vi "LDA2_Safety.vi"(1 "Adam Loop Count":i32, 2 "Ch Names":string[](array[string]), 3 "Values":dbl[](array[numeric]) format="%.2f") -> (0 "Scan comment":string)   [LabVIEW 2015]
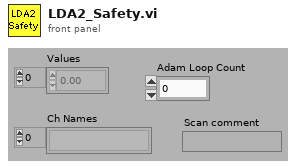
[diagram p1: front panel]
types:
  T1 = typedef "LVDateTimeRec.ctl" = cluster{"fractional second":dbl, "second":i32, "minute":i32, "hour":i32, "day of month":i32, "month":i32, "year":i32, "day of week":i32, "day of year":i32, "DST":i32}
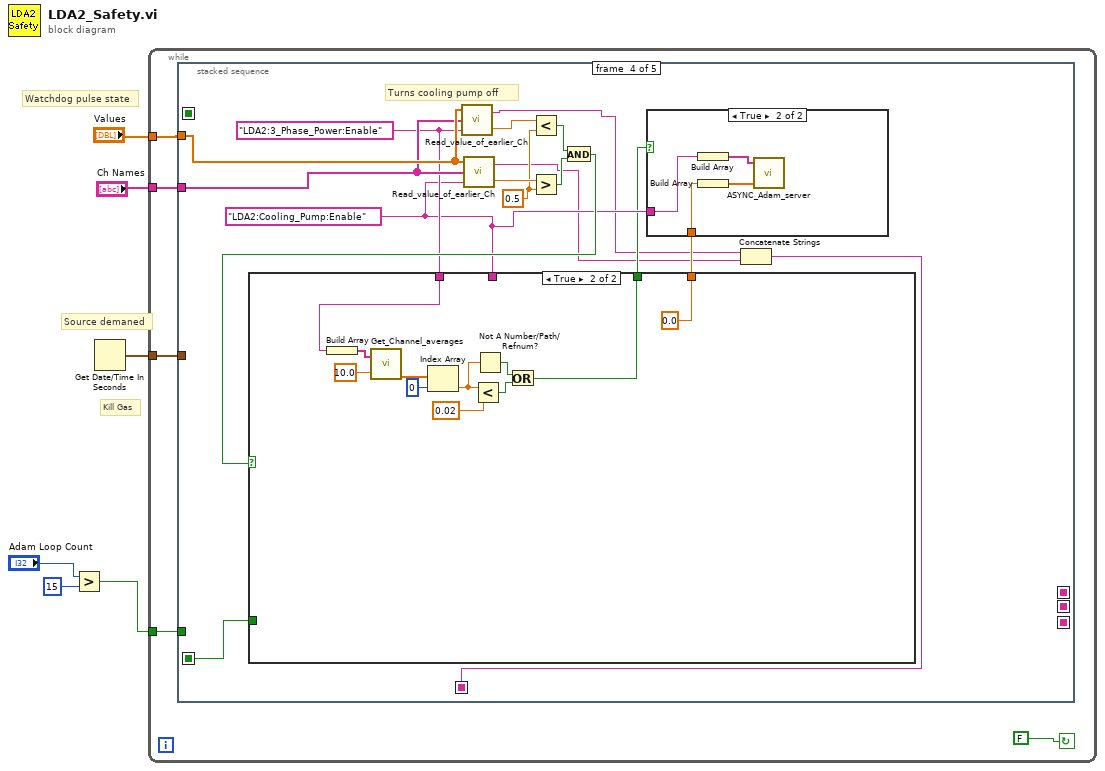
[diagram p0: block diagram]
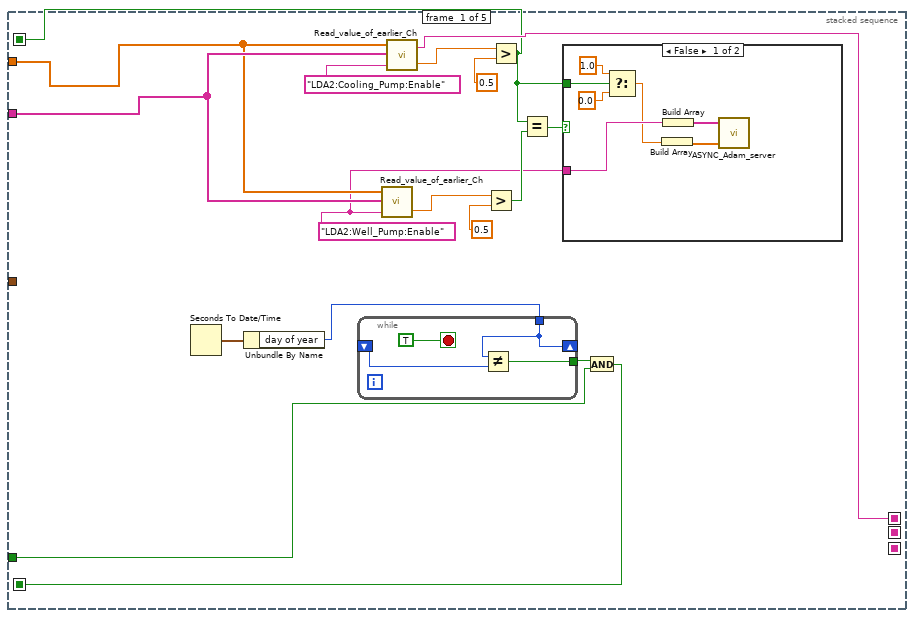
[diagram p2: hidden frame]
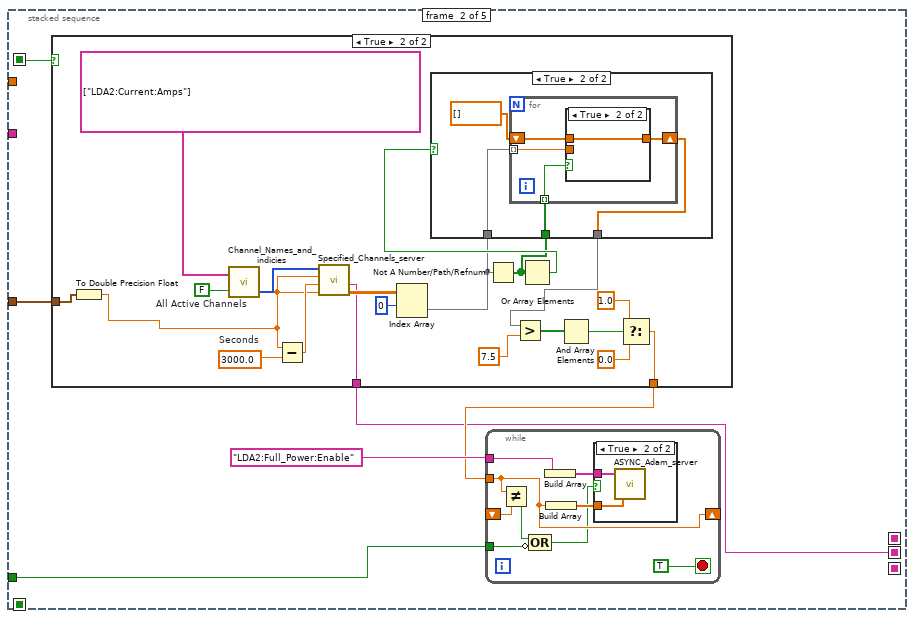
[diagram p4: hidden frame]
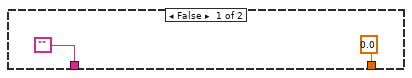
[diagram p6: hidden frame]
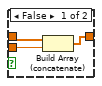
[diagram p8: hidden frame]
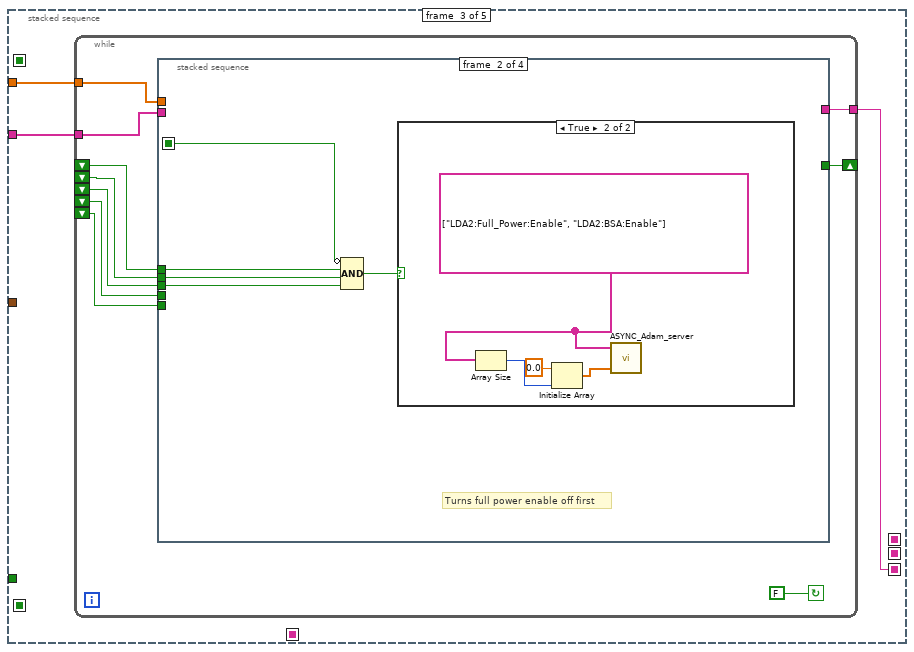
[diagram p9: hidden frame]
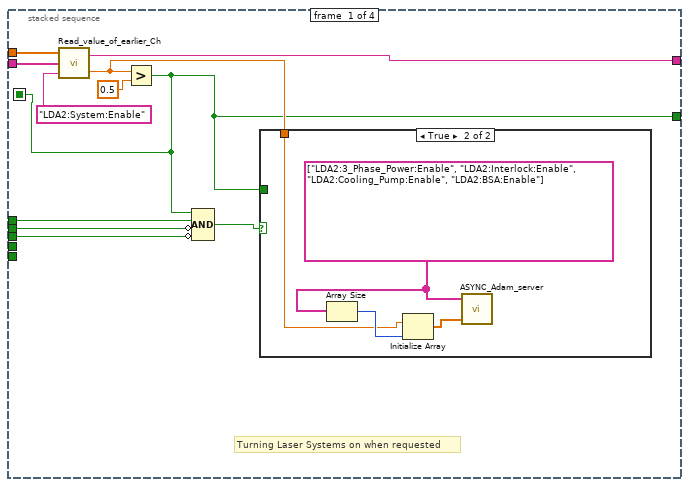
[diagram p10: hidden frame]
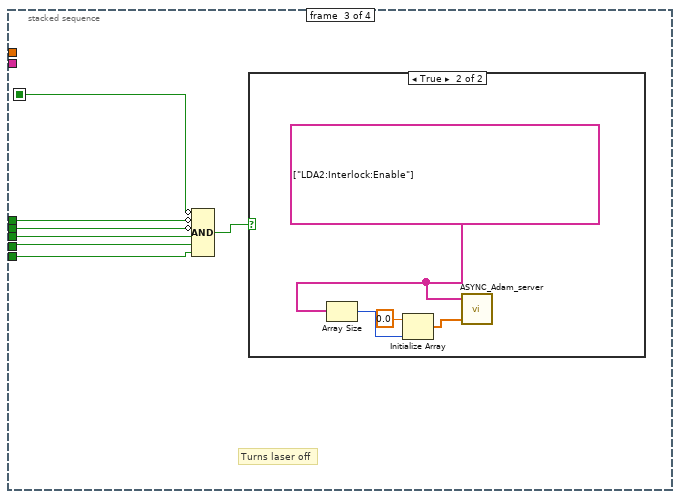
[diagram p13: hidden frame]
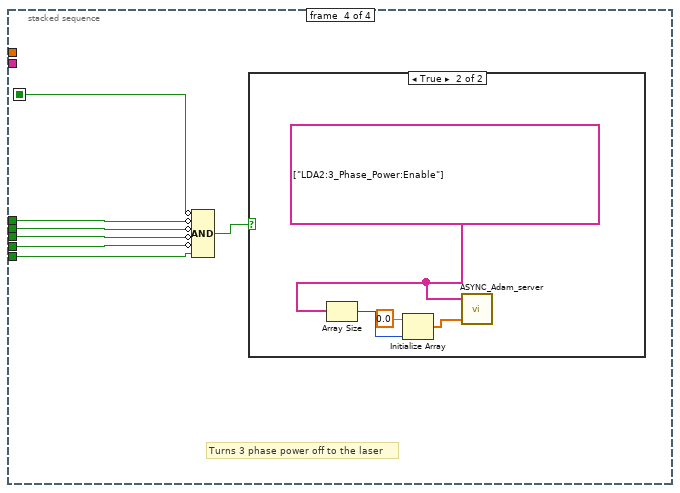
[diagram p15: hidden frame]
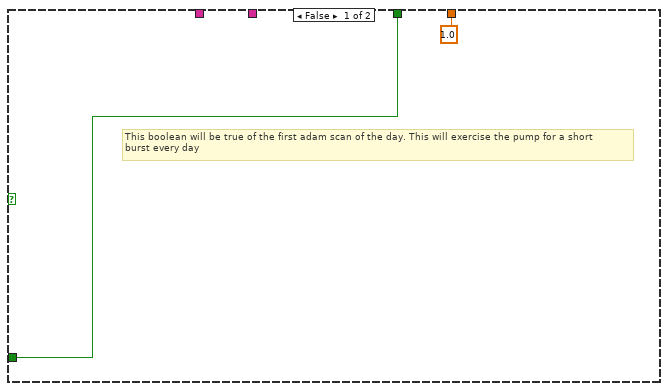
[diagram p18: hidden frame]
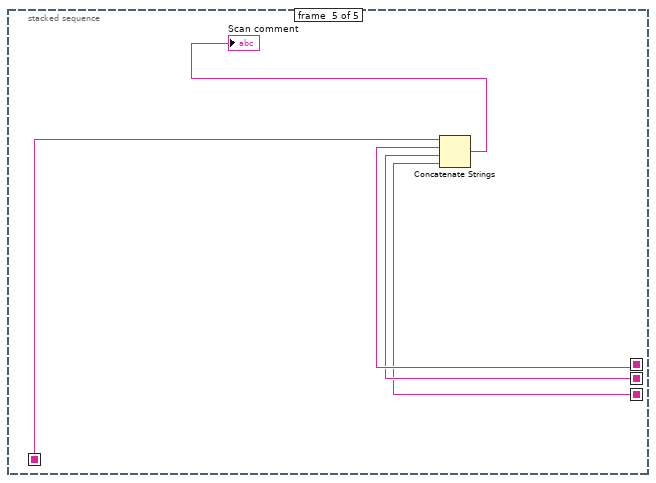
[diagram p19: hidden frame]
diagram:
  # "Source demaned"
  # "Watchdog pulse state"
  # "Kill Gas"
  n1 = Greater?(x="Adam Loop Count", y=15) -> (0:w2:bool)
  n2 = Get Date/Time In Seconds() -> (seconds since 1Jan1904=w1:timestamp)
  n3 = while {
    tunnel: "Ch Names" -> [w11]
    tunnel: "Values" -> [w10]
    tunnel: w2 -> [w8]
    tunnel: w1 -> [w7]
    stop <- FALSE continue-if-true
    n4 = stacked-sequence {
      seq-local: [w21 _ _ _ _] -> [_ _ _ w154 _]
      seq-local: [w12 _ _ _ _] -> [_ w44 _ _ _]
      seq-local: [w25 _ _ _ _] -> [_ _ _ _ w188]
      seq-local: [_ w40 _ _ _] -> [_ _ _ _ w187]
      seq-local: [_ _ w92 _ _] -> [_ _ _ _ w186]
      seq-local: [_ _ _ w151 _] -> [_ _ _ _ w184]
      tunnel: w11 -> [w17 _ w93 w164 _]
      tunnel: w10 -> [w16 _ w94 w165 _]
      tunnel: w8 -> [w20 w42 _ _ _]
      tunnel: w7 -> [_ w45 _ _ _]
      frame #0 {
        w13 = "LDA2:Well_Pump:Enable" ("Desired Ch to Read")
        n5 = Seconds To Date/Time() -> (date time rec=w24:T1)  [unwired: 2 in]
        n6 = Unbundle By Name(w24) -> ("day of year"=w23:i32)
        n7 = while {
          shift-right: [w39] -> _
          shift-left: _ -> [w38]
          tunnel: w23 -> [w39]
          tunnel: [w37] -> w22
          stop <- TRUE stop-if-true
          n8 = Not Equal?(x=w39, y=w38) -> (x != y?=w37:bool)
        }
        n9 = call "Read_value_of_earlier_Ch.vi"("Desired Ch to Read"=w13, "Ch names"=w17, "Present scan array"=w16) -> ("Value"=w18:dbl)  [unwired: 1 in, 1 out]
        n10 = call "Read_value_of_earlier_Ch.vi"("Desired Ch to Read"="LDA2:Cooling_Pump:Enable", "Ch names"=w17, "Present scan array"=w16) -> ("Value"=w27:dbl, "Scan comment"=w25:string)  [unwired: 1 in]
        n11 = Greater?(x=w18, y=0.5) -> (0:w15:bool)
        n12 = Greater?(x=w27, y=0.5) -> (0:w12:bool)
        n13 = Equal?(x=w12, y=w15) -> (x = y?=w14:bool)
        n14 = case shown="False" w14 {
          tunnel: w13 -> [w34 _]
          tunnel: w12 -> [w33 _]
          frame False {
            n15 = Select(t=1.0, s=w33, f=0.0) -> (s? t:f=w30:dbl)
            n16 = Build Array(w30) -> (w29:dbl[])
            n17 = Build Array(w34) -> (w35:string[])
            n18 = call "ASYNC_Adam_server.vi"("Values"=w29, "Channel Names"=w35) -> ()  [unwired: 1 in, 3 out]
          }
          frame True {
          }
        }
        n19 = And(x=w22, y=w20) -> (x .and. y?=w21:bool)
      }
      frame #1 {
        n20 = case shown="True" w44 {
          tunnel: w45 -> [_ w78]
          tunnel: [0.0 ("y") w66] -> w41
          tunnel: ["" w60] -> w40
          frame False {
          }
          frame True {
            w76 = 3000.0  # Seconds
            w74 = FALSE  # All Active Channels
            n21 = To Double Precision Float(number=w78) -> (double precision float=w72:dbl)
            n22 = call "Channel_Names_and_indicies.vi"("All Active Channels"=w74, "Desired Ch Names"=string[] ["LDA2:Current:Amps"]) -> ("Indicies"=w75:i32[])  [unwired: 1 out]
            n23 = Subtract(x=w72, y=w76) -> (x-y=w77:dbl)
            n24 = call "Specified_Channels_server.vi"("End time"=w72, "Start time"=w77, "Clients time"=w72, "Requested channels"=w75) -> ("Output array"=w70:dbl[][], "Messages"=w60:string)  [unwired: 1 in, 3 out]
            n25 = Index Array(array=w70, index (row)=0) -> (element=w59:dbl[])  [unwired: 1 in]
            n26 = Not A Number/Path/Refnum?(number/path/refnum=w59) -> (NaN/Path/Refnum?=w62:bool[])
            n27 = Or Array Elements(Boolean array=w62) -> (logical OR=w63:bool)
            n28 = case shown="True" w63 {
              tunnel: w62 -> [_ w83]
              tunnel: w59 -> [w79 w82]
              tunnel: [w79 w80] -> w61
              frame False {
              }
              frame True {
                n29 = for {
                  shift-right: [w86] -> w80
                  shift-left: dbl[] [] -> [w85]
                  tunnel: w83 -> [w87] mode=indexing
                  tunnel: w82 -> [w84] mode=indexing
                  n30 = case shown="True" w87 {
                    tunnel: [w89 w91] -> w86
                    tunnel: w85 -> [w90 w91]
                    tunnel: w84 -> [w88 _]
                    frame False {
                      n31 = Build Array (concatenate)(w90, w88) -> (w89:dbl[])
                    }
                    frame True {
                    }
                  }
                }
              }
            }
            n32 = Greater?(x=w61, y=7.5) -> (0:w65:bool[])
            n33 = And Array Elements(Boolean array=w65) -> (logical AND=w64:bool)
            n34 = Select(t=1.0 ("y"), s=w64, f=0.0 ("y")) -> (s? t:f=w66:dbl)
          }
        }
        n35 = while {
          shift-right: [w50] -> _
          shift-left: _ -> [w51]
          tunnel: w41 -> [w50]
          tunnel: "LDA2:Full_Power:Enable" -> [w52]
          tunnel: w42 -> [w47]
          stop <- TRUE stop-if-true
          n36 = Not Equal?(x=w50, y=w51) -> (x != y?=w48:bool)
          n37 = Compound Arithmetic op=OR(w48, invert w47) -> (w46:bool)
          n38 = Build Array(w52) -> (w53:string[])
          n39 = Build Array(w50) -> (w54:dbl[])
          n40 = case shown="True" w46 {
            tunnel: w54 -> [_ w56]
            tunnel: w53 -> [_ w55]
            frame False {
            }
            frame True {
              n41 = call "ASYNC_Adam_server.vi"("Values"=w56, "Channel Names"=w55) -> ()  [unwired: 1 in, 3 out]
            }
          }
        }
      }
      frame #2 {
        n42 = while {
          tunnel: w94 -> [w104]
          tunnel: w93 -> [w103]
          shift-right: [w98] -> _
          shift-left: _ -> [w101]
          shift-left: _ -> [w100]
          shift-left: _ -> [w99]
          tunnel: [w97] -> w92
          shift-left: _ -> [w96]
          shift-left: _ -> [w95]
          stop <- FALSE continue-if-true
          n43 = stacked-sequence {
            seq-local: [w106 _ _ _] -> [_ w121 w132 w143]
            tunnel: w104 -> [w115 _ _ _]
            tunnel: w103 -> [w114 _ _ _]
            tunnel: w101 -> [w110 w124 w135 w146]
            tunnel: w100 -> [w109 w123 w134 w145]
            tunnel: w99 -> [w108 w122 w133 w144]
            tunnel: [w106 _ _ _] -> w98
            tunnel: [w107 _ _ _] -> w97
            tunnel: w96 -> [_ _ w130 w141]
            tunnel: w95 -> [_ _ w129 w140]
            frame #0 {
              # "Turning Laser Systems on when requested"
              n44 = call "Read_value_of_earlier_Ch.vi"("Desired Ch to Read"="LDA2:System:Enable", "Ch names"=w114, "Present scan array"=w115) -> ("Value"=w111:dbl, "Scan comment"=w107:string)  [unwired: 1 in]
              n45 = Greater?(x=w111, y=0.5) -> (0:w106:bool)
              n46 = Compound Arithmetic op=AND(w106, w110, invert w109, invert w108) -> (w105:bool)
              n47 = case shown="True" w105 {
                tunnel: w111 -> [_ w116]
                tunnel: w106 -> [_ _]
                frame False {
                }
                frame True {
                  w119 = string[] ["LDA2:3_Phase_Power:Enable", "LDA2:Interlock:Enable", "LDA2:Cooling_Pump:Enable", "LDA2:BSA:Enable"] ("Channel Names")
                  n48 = Array Size(array=w119) -> (size(s)=w117:i32)
                  n49 = Initialize Array(w116, w117) -> (w118:dbl[])
                  n50 = call "ASYNC_Adam_server.vi"("Values"=w118, "Channel Names"=w119) -> ()  [unwired: 1 in, 3 out]
                }
              }
            }
            frame #1 {
              # "Turns full power enable off first"
              n51 = Compound Arithmetic op=AND(invert w121, w124, w123, w122) -> (w120:bool)
              n52 = case shown="True" w120 {
                frame False {
                }
                frame True {
                  w125 = string[] ["LDA2:Full_Power:Enable", "LDA2:BSA:Enable"] ("Channel Names")
                  n53 = Array Size(array=w125) -> (size(s)=w127:i32)
                  n54 = Initialize Array(0.0, w127) -> (w128:dbl[])
                  n55 = call "ASYNC_Adam_server.vi"("Values"=w128, "Channel Names"=w125) -> ()  [unwired: 1 in, 3 out]
                }
              }
            }
            frame #2 {
              # "Turns laser off"
              n56 = Compound Arithmetic op=AND(invert w132, invert w135, invert w134, w133, w130, w129) -> (w131:bool)
              n57 = case shown="True" w131 {
                frame False {
                }
                frame True {
                  w136 = string[] ["LDA2:Interlock:Enable"] ("Channel Names")
                  n58 = Array Size(array=w136) -> (size(s)=w138:i32)
                  n59 = Initialize Array(0.0, w138) -> (w139:dbl[])
                  n60 = call "ASYNC_Adam_server.vi"("Values"=w139, "Channel Names"=w136) -> ()  [unwired: 1 in, 3 out]
                }
              }
            }
            frame #3 {
              # "Turns 3 phase power off to the laser"
              n61 = Compound Arithmetic op=AND(invert w143, invert w146, invert w145, invert w144, invert w141, w140) -> (w142:bool)
              n62 = case shown="True" w142 {
                frame False {
                }
                frame True {
                  w147 = string[] ["LDA2:3_Phase_Power:Enable"] ("Channel Names")
                  n63 = Array Size(array=w147) -> (size(s)=w149:i32)
                  n64 = Initialize Array(0.0, w149) -> (w150:dbl[])
                  n65 = call "ASYNC_Adam_server.vi"("Values"=w150, "Channel Names"=w147) -> ()  [unwired: 1 in, 3 out]
                }
              }
            }
          }
        }
      }
      frame #3 {
        w158 = "LDA2:3_Phase_Power:Enable" ("Desired Ch to Read")
        w163 = 0.5 ("y")
        w157 = "LDA2:Cooling_Pump:Enable" ("Desired Ch to Read")
        # "Turns cooling pump off"
        n66 = call "Read_value_of_earlier_Ch.vi"("Desired Ch to Read"=w158, "Ch names"=w164, "Present scan array"=w165) -> ("Value"=w162:dbl, "Scan comment"=w153:string)  [unwired: 1 in]
        n67 = call "Read_value_of_earlier_Ch.vi"("Desired Ch to Read"=w157, "Ch names"=w164, "Present scan array"=w165) -> ("Value"=w166:dbl, "Scan comment"=w152:string)  [unwired: 1 in]
        n68 = Less?(x=w162, y=w163) -> (x < y?=w161:bool)
        n69 = Greater?(x=w166, y=w163) -> (0:w160:bool)
        n70 = And(x=w161, y=w160) -> (x .and. y?=w159:bool)
        n71 = case shown="True" w159 {
          tunnel: w158 -> [_ w178]
          tunnel: w157 -> [_ _]
          tunnel: [w171 w173] -> w156
          tunnel: [1.0 ("element") 0.0 ("element")] -> w155
          tunnel: w154 -> [w171 _]
          frame False {
            # "This boolean will be true of the first adam scan of the day. This will exercise the pump for a short\nburst every day"
          }
          frame True {
            n72 = Build Array(w178) -> (w182:string[])
            n73 = call "Get_Channel_averages.vi"("Desired Ch Names"=w182, "Averaging time (mins)"=10.0) -> ("number"=w181:dbl[])  [unwired: 1 in, 2 out]
            n74 = Index Array(array=w181, index=0) -> (element=w176:dbl)
            n75 = Less?(x=w176, y=0.02) -> (x < y?=w175:bool)
            n76 = Not A Number/Path/Refnum?(number/path/refnum=w176) -> (NaN/Path/Refnum?=w174:bool)
            n77 = Or(x=w174, y=w175) -> (x .or. y?=w173:bool)
          }
        }
        n78 = case shown="True" w156 {
          tunnel: w157 -> [_ w168]
          tunnel: w155 -> [_ w167]
          frame False {
          }
          frame True {
            n79 = Build Array(w168) -> (w169:string[])
            n80 = Build Array(w167) -> (w170:dbl[])
            n81 = call "ASYNC_Adam_server.vi"("Values"=w170, "Channel Names"=w169) -> ()  [unwired: 1 in, 3 out]
          }
        }
        n82 = Concatenate Strings(w153, w152) -> (w151:string)
      }
      frame #4 {
        n83 = Concatenate Strings(w184, w188, w187, w186) -> (→"Scan comment":string)
      }
    }
  }
